vi "CAN Transmit Loop.vi"(9 "LowPriorityQueue":T1, 11 "HighPriorityQueue":T1) -> ()   [LabVIEW 2015]
uses:
  CAN Message Queue.ctl
  CAN Message.ctl
  Global Data.vi
  <vilib>/RioEmbeddedCAN/RioEmbeddedCAN.llb/CANWaitTransmitComplete.vi
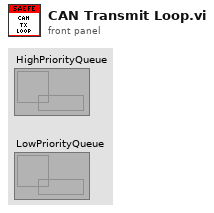
[diagram p1: front panel]
types:
  T1 = typedef "CAN Message Queue.ctl" = refnum<k33>
  T2 = typedef "CAN Message.ctl" = cluster{"identifier":u32, "extended?":bool, "type":u8, "data":cluster{"B0":u8, "B1":u8, "B2":u8, "B3":u8, "B4":u8, "B5":u8, "B6":u8, "B7":u8}}
  T3 = typedef "CANFrameControl.ctl" = cluster{"identifier":u32, "extended?":bool, "type":u8, "payload":u8[]}
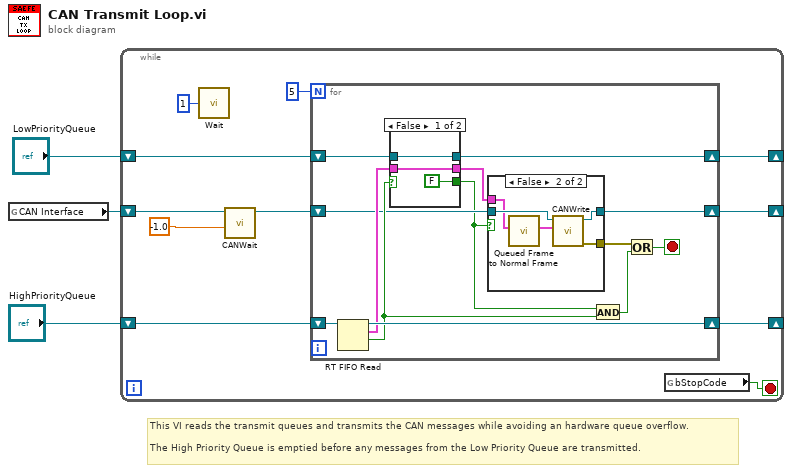
[diagram p0: block diagram]
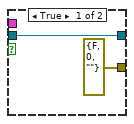
[diagram p2: hidden frame]
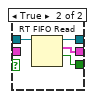
[diagram p3: hidden frame]
diagram:
  # "This VI reads the transmit queues and transmits the CAN messages while avoiding an hardware queue overflow.\n\nThe High Priority Queue is emptied before any messages from the Low Priority Queue are transmitted."
  n1 = global read "Global Data.vi" "CAN Interface"() -> (w1:refnum<k20>)
  n2 = while {
    shift-right: [w6] -> _
    shift-left: "HighPriorityQueue" -> [w8]
    shift-right: [w5] -> _
    shift-left: "LowPriorityQueue" -> [w7]
    shift-right: [w9] -> _
    shift-left: w1 -> [w13]
    stop <- w14 stop-if-true
    n3 = call "Wait"("Count(mSec)"=u32 1) -> ()  [unwired: 1 out]
    n4 = call-poly <vilib>:"CANWait.vi"("timeout (0 s)"=-1.0, "interface object in"=w13) -> ("interface object out"=w10:refnum<k20>)  [unwired: 8 in, 1 out]
    n5 = for {
      N: 5 -> [_]
      shift-right: [w21] -> w9
      shift-left: w10 -> [w17]
      shift-right: [w26] -> w6
      shift-left: w8 -> [w27]
      shift-right: [w24] -> w5
      shift-left: w7 -> [w25]
      stop <- w20 stop-if-true
      n6 = RT FIFO Read(0:w27) -> (8:w26:T1, 9:w22:T2, 10:w23:bool)  [unwired: 3 in, 2 out]
      n7 = case shown="False" w23 {
        tunnel: w25 -> [w37 w41]
        tunnel: [w37 w40] -> w24
        tunnel: [FALSE ("empty?") w39] -> w16
        tunnel: w22 -> [w35 _]
        tunnel: [w35 w38] -> w15
        frame False {
        }
        frame True {
          n8 = RT FIFO Read(0:w41) -> (8:w40:T1, 9:w38:T2, 10:w39:bool)  [unwired: 3 in, 2 out]
        }
      }
      n9 = case shown="False" w16 {
        tunnel: [w29 w34] -> w21
        tunnel: [errorcluster {"status"=FALSE, "code"=0, "source"=""} ("error out") w33] -> w18
        tunnel: w17 -> [w29 w32]
        tunnel: w15 -> [_ w30]
        frame True {
        }
        frame False {
          n10 = call "Queued Frame to Normal Frame.vi"("CAN frame in"=w30) -> ("CAN frame out"=w31:T3)  [unwired: 10 in]
          n11 = call <vilib>:"CANWrite.vi"("CAN frame"=w31, "interface object in"=w32) -> ("error out"=w33:errorcluster, "interface object out"=w34:refnum<k20>)  [unwired: 8 in]
        }
      }
      n12 = And(x=w16, y=w23) -> (x .and. y?=w19:bool)
      n13 = Or(x=w18, y=w19) -> (x .or. y?=w20:bool)
    }
    n14 = global read "Global Data.vi" "bStopCode"() -> (w14:bool)
  }
